vi "systemtime_to_string.vi"(10 "time format string (%c)":string="%c", 11 "UTC Date and Time in":T1={"Year"=0, "Month"=1, "DayOfWeek"=0, "Day"=0, "Hour"=0, "Minute"=0, "Seconds"=0, "Milliseconds"=0} {"DayOfWeek" items=["Sunday", "Monday", "Tuesday", "Wednesday", "Thursday", "Friday", "Saturday"]; "Month" items=["", "January", "February", "March", "April", "May", "June", "July", "August", "September", "October", "November", "December"]}) -> (3 "UTC Date and Time out (string)":string)   [LabVIEW 2010]
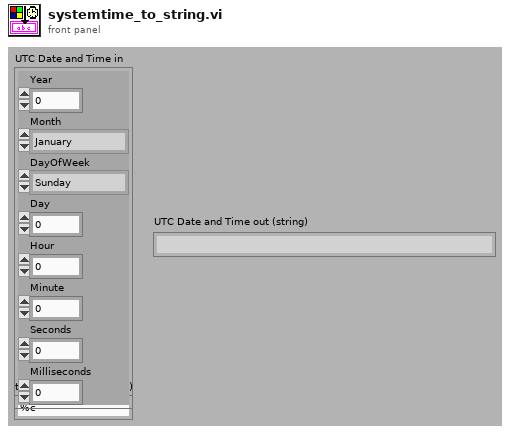
[diagram p1: front panel]
types:
  T1 = cluster{"Year":u16, "Month":u16, "DayOfWeek":u16, "Day":u16, "Hour":u16, "Minute":u16, "Seconds":u16, "Milliseconds":u16}
  T2 = cluster{"Seconds":i32, "Minute":i32, "Hour":i32, "Day":i32, "Month":i32, "Year":i32, "DayOfWeek":i32, i32, i32}
  T3 = cluster{"Year":i32, "Month":i32, "DayOfWeek":i32, "Day":i32, "Hour":i32, "Minute":i32, "Seconds":i32, "Milliseconds":i32}
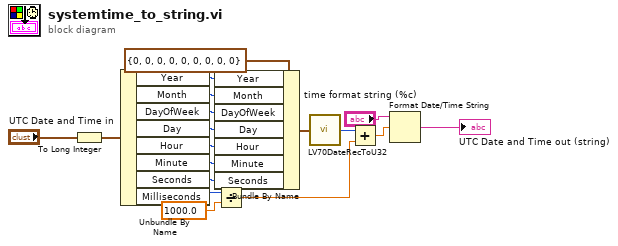
[diagram p0: block diagram]
diagram:
  n1 = To Long Integer(number="UTC Date and Time in") -> (32bit integer=w2:T3)
  n2 = Unbundle By Name(w2) -> ("Year"=w4:i32, "Month"=w10:i32, "DayOfWeek"=w8:i32, "Day"=w9:i32, "Hour"=w7:i32, "Minute"=w6:i32, "Seconds"=w5:i32, "Milliseconds"=w12:i32)
  n3 = Bundle By Name(cluster=T2 {"Seconds"=0, "Minute"=0, "Hour"=0, "Day"=0, "Month"=0, "Year"=0, "DayOfWeek"=0, 0, 0} ("output cluster"), "Year"=w4, "Month"=w10, "DayOfWeek"=w8, "Day"=w9, "Hour"=w7, "Minute"=w6, "Seconds"=w5) -> (w11:T2)
  n4 = Divide(x=w12, y=1000.0) -> (x/y=w15:dbl)
  n5 = call <vilib>:"LV70DateRecToU32.vi"("date time rec"=w11) -> ("Time"=w14:u32)
  n6 = Add(x=w14, y=w15) -> (x+y=w16:dbl)
  n7 = Format Date/Time String(time format string (%c)="time format string (%c)", seconds (now)=w16) -> (date/time string=→"UTC Date and Time out (string)":string)  [unwired: 1 in]
